vi "XY Graph Get TipStrip Visible.vi"(8 "Error In":errorcluster, 10 "TipStrip Visible":bool, 11 "XYGraph Refnum":T1) -> (0 "Error Out":errorcluster, 1 "TipStrip Visible Found?":bool, 2 "TipStrip Visible":bool, 3 "XYGraph Refnum":T1)   [LabVIEW 2021, in "XY Graph Add-Ons.lvlib"]
uses:
  XY Graph Add-Ons.lvlib
  XY Graph Refnum.ctl
  XY Graph Property Tag List.ctl
  c650eaaa-2c64-4f1d-a897-450eefccb08a.vi
  Variant/Variant to Data/Variant to Boolean.vi
  <vilib>/UserTags/UserTags.lvlib
  Variant/Variant to Data/Variant to Data.lvlib
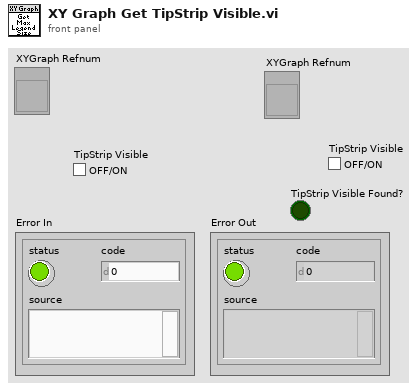
[diagram p1: front panel]
types:
  T1 = typedef "XY Graph Add-Ons.lvlib/XY Graph Refnum.ctl" = refnum<vi>
  T2 = typedef "XY Graph Add-Ons.lvlib/XY Graph Property Tag List.ctl" = enum16{"Max Legend Size", "Preserved Plots", "XScales.GridColors", "YScales.GridColors", "TipStrip String", "TipStrip Visible", "Tool Panels Visibility", "Plots Metadata"}
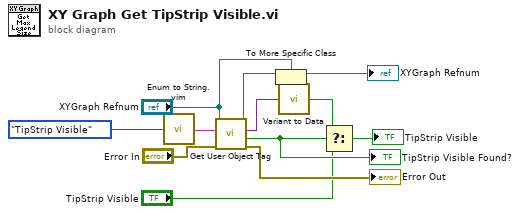
[diagram p0: block diagram]
diagram:
  n1 = call "Enum to String.vim"("Enum"=XY_Graph_Property_Tag_List."TipStrip Visible" ("XY Graph Property Tag")) -> ("String"=w1:string)
  n2 = call <vilib>:"Get User Object Tag.vi"("error in (no error)"="Error In", "Tag Name"=w1, "Generic Refnum"="XYGraph Refnum") -> ("error out"=→"Error Out":errorcluster, "Was Tag Found?"=w7:bool, "Value"=w10:variant, "dup Generic Refnum"=w5:refnum<vi>)  [unwired: 5 in]
  "TipStrip Visible Found?" <- w7
  n3 = To More Specific Class(target class="XYGraph Refnum", reference=w5) -> (specific class reference=→"XYGraph Refnum":T1)  [unwired: 1 in, 1 out]
  n4 = call-poly "Variant to Data.vi"("Variant"=w10) -> ("Value"=w9:bool)  [unwired: 8 in]
  n5 = Select(t=w9, s=w7, f="TipStrip Visible") -> (s? t:f=→"TipStrip Visible":bool)
